vi "Process-Fire occurrence.vi"(10 "Abort logging":bool, 11 "Wait on post-processing":refnum<k4>) -> ()   [LabVIEW 2020]
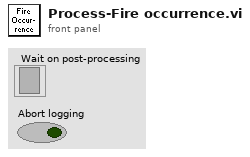
[diagram p1: front panel]
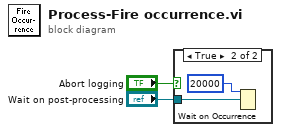
[diagram p0: block diagram]
diagram:
  n1 = case shown="True" "Abort logging" {
    tunnel: "Wait on post-processing" -> [_ w3]
    frame False {
    }
    frame True {
      n2 = Wait on Occurrence(2:w3, 3:20000 ("ms timeout (-1)")) -> ()  [unwired: 1 in, 1 out]
    }
  }
